vi "Write receiverTacticState .vi"(8 "error in (no error)":errorcluster, 10 "tactic":T1, 11 "PassTactic in":refnum<class "PassTactic.lvclass">) -> (0 "error out":errorcluster, 3 "PassTactic out":refnum<class "PassTactic.lvclass">)   [LabVIEW 2023, in "PassTactic.lvclass"]
uses:
  PassTactic.lvclass
  Robot_class/tactics.ctl
  PassTactic.lvclass/PassTactic.ctl
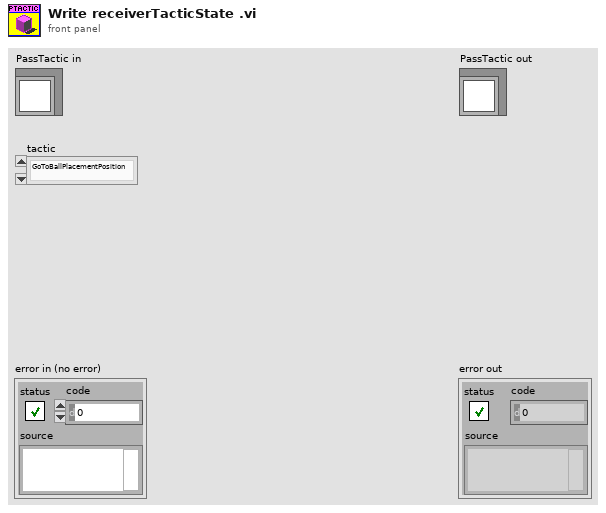
[diagram p1: front panel]
types:
  T1 = typedef "tactics.ctl" = enum16{"GoToBallPlacementPosition", "PlaceBall", "GoToBallPlacement", "5Robots", "BallPlacementEnemy", "ReceivePassInFuturePoint", "Roller", "PrepareRollToPassRollerGoTo", "PrepareRollToPassReceiverGoTo", "WaitRoll", "PositionToRoll", "PenaltyAttacker", "PassObserver", "PenaltyDefense", "TableReceiverTactic", "Test", "DefendGoal", "Marker", "FollowAttacker", "DefendArea", "Shoot", "AttackerAimGoal", "AttackerBallOutOfField", "AttackerBlock", "AttackerStop", "Duelist", "Halt", "ZigZag", "GoTo", "Timeout", "KickToBestRobot", "KickToPassReceiver", "PositionToReceivePass", "WaitPass"}
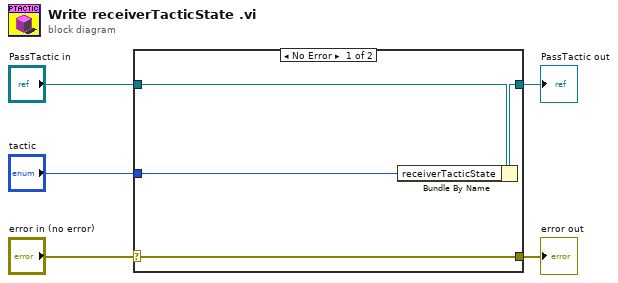
[diagram p0: block diagram]
diagram:
  n1 = case shown="No Error" "error in (no error)" {
    selector: "error in (no error)" -> [w9 w10]
    tunnel: [w9 w10] -> w4
    tunnel: [w7 w11] -> w2
    tunnel: "PassTactic in" -> [w8 w11]
    tunnel: "tactic" -> [w6 _]
    frame No Error {
      n2 = Bundle By Name(cluster=w8, "receiverTacticState"=w6) -> (w7:refnum<class "PassTactic.lvclass">)
    }
    frame Error {
    }
  }
  "error out" <- w4
  "PassTactic out" <- w2
